vi "snapdragon_elka_quad.vi"() -> ()   [LabVIEW 2017]
uses:
  <vilib>/Instr/_visa.llb/VISA Flush IO Buffer Mask.ctl
  <vilib>/Instr/_visa.llb/VISA Configure Serial Port (Instr).vi
  <vilib>/Utility/file.llb/Write Delimited Spreadsheet (I64).vi
panel:
  in  "vio_yawki":i16=192
  in  "ixy_sens":i16=41
  in  "vio_yawkp":i16=2322
  in  "z_ki":i16=188
  out "base_thrust":i16(graph)
  in  "file path (dialog if empty) 2":path=path "C:/Users/Eric Solomon/Documents/elka/tests/sample_test.txt"
  in  "writte to file? 2":bool
  out "roll":i32(graph)
  out "thrust":i32(graph)
  out "z_error":i32(graph)
  out "y_error":i32(graph)
  in  "alt_kd":i16=-2
  in  "alt_kp":i16=-4
  in  "z_kp":i16=2330
  in  "z_kd":i16=70
  in  "vxy_sens":i16=26
  in  "xy_sens":i16=122
  in  "yawkd":i16=80
  in  "rollki":i16
  in  "rollkp":i16=2
  in  "Thrust Trim":i16(slide)=900 scale=-200.0..1500.0
  in  "Roll Trim":i16(slide) scale=-1000.0..1000.0
  in  "Pitch Trim":i16(slide) scale=-1000.0..1000.0
  in  "Yaw Trim":i16(slide) scale=-2000.0..2000.0
  out "appended array 2":u32[](array[numeric])=[11, 3, 255, 255, 3, 132, 0, 0, 0, 0, 0, 0]
  out "read buffer 2":string
  in  "STOP TRIM":bool
  out "read buffer 4":string
  out "appended array 4":u32[](array[numeric])=[15, 2, 255, 255, 0, 10, 0, 2, 0, 2, 255, 246, 255, 252, 255, 254]
  in  "Yaw_sens":i16=-10
  in  "Pitch_sens":i16=2
  in  "Roll_sens":i16=2
  in  "Thrust_sens":i16=10
  out "read buffer 3":string
  out "appended array 3":u32[](array[numeric])=[25, 1, 255, 255, 0, 2, 0, 0, 0, 40, 0, 2, 0, 0, 0, 40, 255, 176, 0, 15, 255, 248, 0, 7, 0, 5]
  in  "rollkd":i16=40
  in  "pitchki":i16
  in  "pitchkd":i16=40
  in  "pitchkp":i16=-2
  out "appended array":u32[](array[numeric])
  in  "channel4":i16
  in  "channel3":i16
  in  "channel2":i16
  in  "channel1":i16(slide) scale=0.0..2000.0
  out "read buffer":string
  out "pilot array":u8[](array[numeric])=[255, 247, 5, 220, 0, 15, 0, 115, 254, 40, 0, 0, 0, 0, 0, 0, 0, 0, 0, 0, 0, 0, 0, 0, 0, 0, 3, 132, 0, 2]
  out "GYRO X (deg/s)":i16(graph)=-9
  out "GYRO Y":i16(graph)=1500
  out "GYRO Z":i16(graph)=15
  out "Roll":i16(graph)=115
  out "Pitch":i16(graph)=-472
  out "x_error":i32(graph)
  out "Serial Settings:Number of Bytes at Serial Port":u32=32
  in  "XBEE STOP":bool
  in  "flow control 3":u16(ring) items=["None"=0, "XON/XOFF"=1, "RTS/CTS"=2, "DTR/DSR"=4]
  in  "stop bits 3":u16(ring)=10 items=["1.0"=10, "1.5"=15, "2.0"=20]
  in  "parity 3":u16(ring) items=["None", "Odd", "Even", "Mark", "Space"]
  in  "data bits 3":u16=8 min=5 max=8 step=1
  in  "VISA resource name 3":refnum<visa-resource-name>="COM7"
  in  "baud rate 3":u32=38400
  # "RECEIVE"
  # "GAINS"
  # "SENSITIVITY"
  # "Attitude Gains"
  # "Position Gains"
  # "-8"
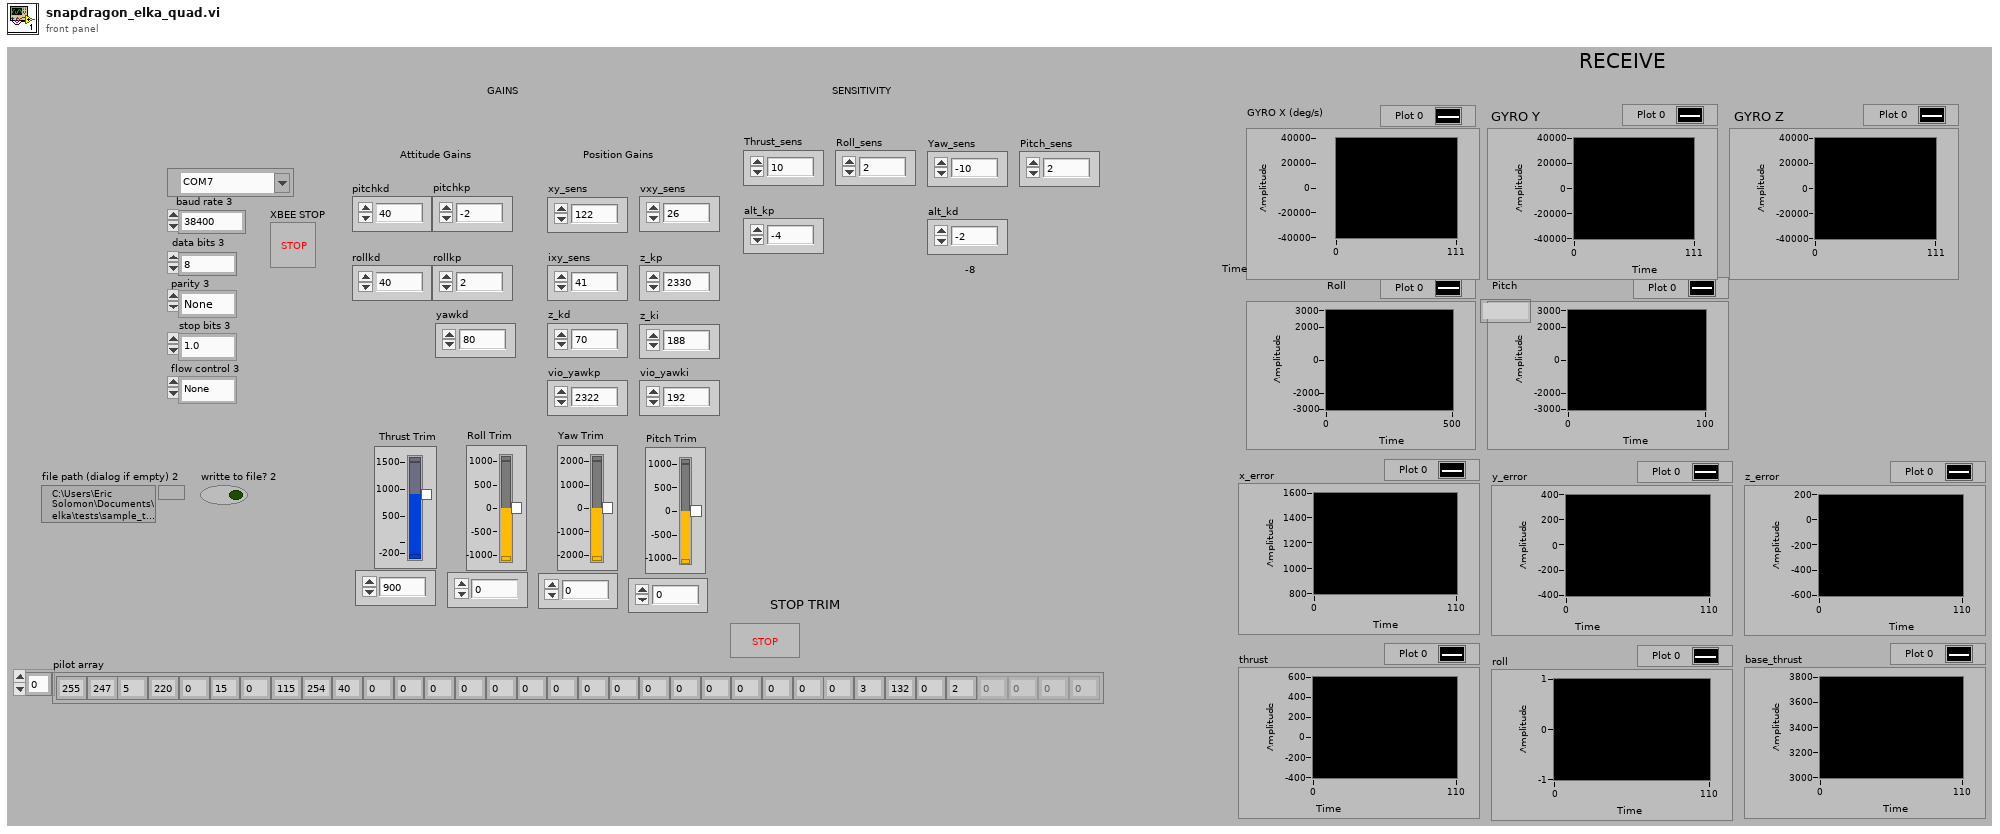
[diagram p1: front panel]
types:
  T1 = cluster{i32, i32, i32, i32, i32, i32, i32, i32, i32, i32, i32, i32, i32, i32, i32, i32}
  T2 = typedef "VISA Flush IO Buffer Mask.ctl" = u16
  T3 = cluster{i16, i16, i16, i16, i16, i32, i32, i32, i32, i32, i16, i32, i32, i32, i32, "millisecond timer value":u32}
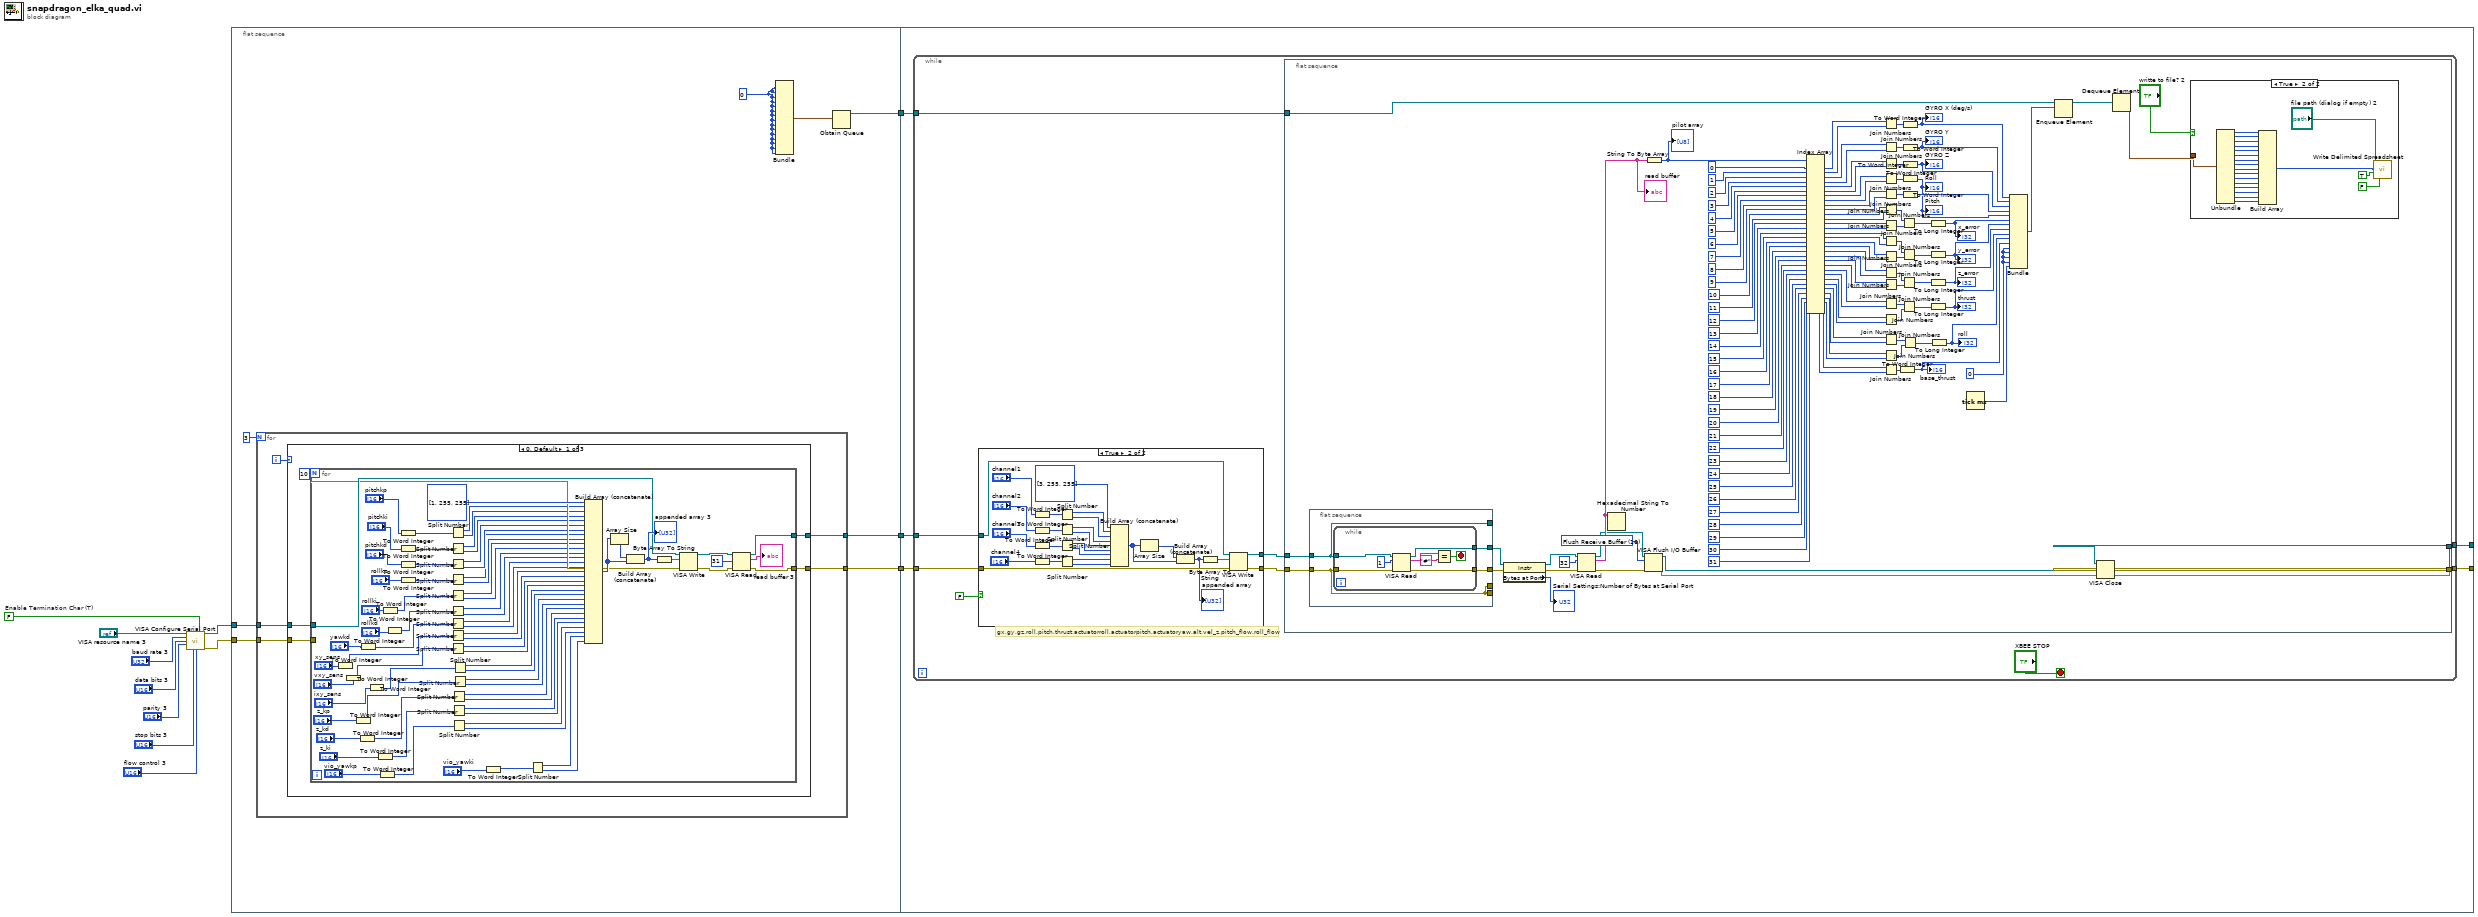
[diagram p0: block diagram]
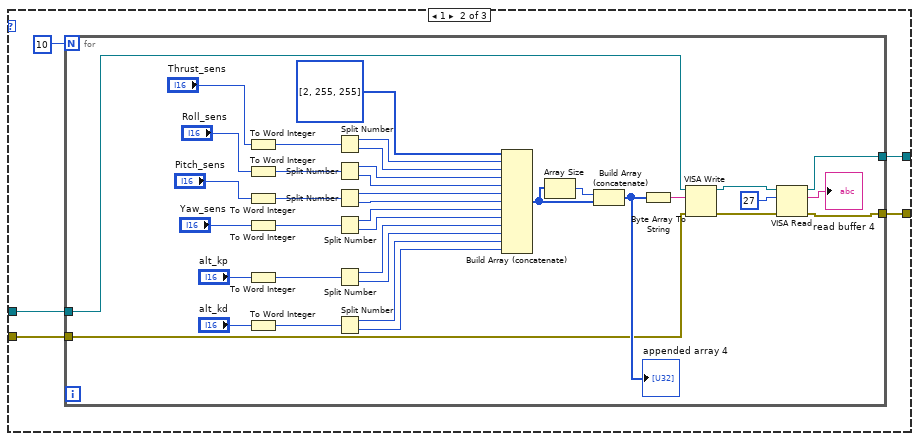
[diagram p2: hidden frame]
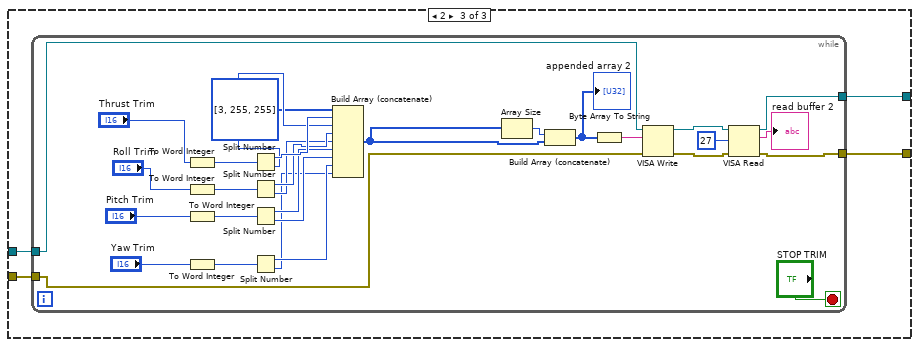
[diagram p3: hidden frame]
diagram:
  w11 = FALSE  # Enable Termination Char (T)
  n1 = call-poly "VISA Configure Serial Port"("VISA resource name"="VISA resource name 3", "Enable Termination\nChar (T)"=w11, "baud rate (9600)"="baud rate 3", "data bits (8)"="data bits 3", "parity (0:none)"="parity 3", "stop bits (10: 1 bit)"="stop bits 3", "flow control (0:none)"="flow control 3") -> ("VISA resource name out"=w6:refnum<visa-resource-name>, "error out"=w5:errorcluster)  [unwired: 1 in, 6 out]
  n2 = flat-sequence {
    tunnel: w5 -> [w21]
    tunnel: w6 -> [w22]
    tunnel: [w20] -> w4
    tunnel: [w19] -> w3
    tunnel: [w15] -> w1
    tunnel: [w186] -> w7
    tunnel: w4 -> [w185]
    tunnel: w3 -> [w184]
    tunnel: [w183] -> w2
    tunnel: w1 -> [w182]
    frame #0 {
      w16 = 0
      n3 = for {
        N: 3 -> [_]
        tunnel: w22 -> [w27]
        tunnel: [w25] -> w20
        tunnel: w21 -> [w26]
        tunnel: [w24] -> w19
        i -> [w23]
        n4 = case shown="0, Default" w23 {
          tunnel: w27 -> [w32 w110 w151]
          tunnel: w26 -> [w31 w107 w150]
          tunnel: [w30 w109 w149] -> w25
          tunnel: [w29 w108 w148] -> w24
          frame 0, Default {
            n5 = for {
              N: 10 -> [_]
              tunnel: w32 -> [w91]
              tunnel: [w89] -> w30
              tunnel: w31 -> [w90]
              tunnel: [w88] -> w29
              n6 = To Word Integer(number="xy_sens") -> (16bit integer=w72:i16)
              n7 = To Word Integer(number="vxy_sens") -> (16bit integer=w71:i16)
              n8 = To Word Integer(number="z_kp") -> (16bit integer=w70:i16)
              n9 = To Word Integer(number="z_kd") -> (16bit integer=w69:i16)
              n10 = To Word Integer(number="yawkd") -> (16bit integer=w84:i16)
              n11 = To Word Integer(number="ixy_sens") -> (16bit integer=w37:i16)
              n12 = To Word Integer(number="z_ki") -> (16bit integer=w58:i16)
              n13 = To Word Integer(number="vio_yawkp") -> (16bit integer=w57:i16)
              n14 = To Word Integer(number="rollki") -> (16bit integer=w86:i16)
              n15 = To Word Integer(number="rollkd") -> (16bit integer=w85:i16)
              n16 = To Word Integer(number="pitchkp") -> (16bit integer=w104:i16)
              n17 = To Word Integer(number="pitchki") -> (16bit integer=w103:i16)
              n18 = To Word Integer(number="pitchkd") -> (16bit integer=w102:i16)
              n19 = To Word Integer(number="rollkp") -> (16bit integer=w101:i16)
              n20 = Split Number(x=w104) -> (hi(x)=w52:u8, lo(x)=w51:u8)
              n21 = Split Number(x=w103) -> (hi(x)=w50:u8, lo(x)=w49:u8)
              n22 = Split Number(x=w102) -> (hi(x)=w48:u8, lo(x)=w47:u8)
              n23 = Split Number(x=w101) -> (hi(x)=w46:u8, lo(x)=w45:u8)
              n24 = Split Number(x=w86) -> (hi(x)=w44:u8, lo(x)=w43:u8)
              n25 = Split Number(x=w85) -> (hi(x)=w42:u8, lo(x)=w41:u8)
              n26 = Split Number(x=w84) -> (hi(x)=w83:u8, lo(x)=w82:u8)
              n27 = Split Number(x=w72) -> (hi(x)=w61:u8, lo(x)=w62:u8)
              n28 = Split Number(x=w71) -> (hi(x)=w63:u8, lo(x)=w64:u8)
              n29 = Split Number(x=w69) -> (hi(x)=w67:u8, lo(x)=w68:u8)
              n30 = Split Number(x=w57) -> (hi(x)=w54:u8, lo(x)=w53:u8)
              n31 = Split Number(x=w58) -> (hi(x)=w56:u8, lo(x)=w55:u8)
              n32 = Split Number(x=w37) -> (hi(x)=w39:u8, lo(x)=w38:u8)
              n33 = Split Number(x=w70) -> (hi(x)=w65:u8, lo(x)=w66:u8)
              n34 = To Word Integer(number="vio_yawki") -> (16bit integer=w34:i16)
              n35 = Split Number(x=w34) -> (hi(x)=w36:u8, lo(x)=w35:u8)
              n36 = Build Array (concatenate)(i32[] [1, 255, 255], w52, w51, w50, w49, w48, w47, w46, w45, w44, w43, w42, w41, w83, w82, w61, w62, w63, w64, w39, w38, w65, w66, w67, w68, w56, w55, w54, w53, w36, w35) -> (w98:i32[])
              n37 = Array Size(array=w98) -> (size(s)=w99:i32)
              n38 = Build Array (concatenate)(w99, w98) -> (w97:i32[])
              "appended array 3" <- w97
              n39 = Byte Array To String(unsigned byte array=w97) -> (string=w100:string)
              n40 = VISA Write(VISA resource name=w91, write buffer=w100, error in (no error)=w90) -> (VISA resource name out=w95:refnum<visa-resource-name>, error out=w94:errorcluster)  [unwired: 1 out]
              n41 = VISA Read(VISA resource name=w95, byte count=u32 31, error in (no error)=w94) -> (VISA resource name out=w89:refnum<visa-resource-name>, read buffer=→"read buffer 3":string, error out=w88:errorcluster)  [unwired: 1 out]
            }
          }
          frame 1 {
            n42 = for {
              N: 10 -> [_]
              tunnel: w110 -> [w122]
              tunnel: [w121] -> w109
              tunnel: w107 -> [w119]
              tunnel: [w120] -> w108
              n43 = To Word Integer(number="Thrust_sens") -> (16bit integer=w146:i16)
              n44 = To Word Integer(number="Roll_sens") -> (16bit integer=w144:i16)
              n45 = To Word Integer(number="Pitch_sens") -> (16bit integer=w142:i16)
              n46 = To Word Integer(number="Yaw_sens") -> (16bit integer=w140:i16)
              n47 = To Word Integer(number="alt_kp") -> (16bit integer=w116:i16)
              n48 = To Word Integer(number="alt_kd") -> (16bit integer=w115:i16)
              n49 = Split Number(x=w146) -> (hi(x)=w139:u8, lo(x)=w138:u8)
              n50 = Split Number(x=w144) -> (hi(x)=w137:u8, lo(x)=w136:u8)
              n51 = Split Number(x=w142) -> (hi(x)=w135:u8, lo(x)=w134:u8)
              n52 = Split Number(x=w140) -> (hi(x)=w133:u8, lo(x)=w132:u8)
              n53 = Split Number(x=w116) -> (hi(x)=w114:u8, lo(x)=w113:u8)
              n54 = Split Number(x=w115) -> (hi(x)=w112:u8, lo(x)=w111:u8)
              n55 = Build Array (concatenate)(i32[] [2, 255, 255], w139, w138, w137, w136, w135, w134, w133, w132, w114, w113, w112, w111) -> (w129:i32[])
              n56 = Array Size(array=w129) -> (size(s)=w130:i32)
              n57 = Build Array (concatenate)(w130, w129) -> (w128:i32[])
              "appended array 4" <- w128
              n58 = Byte Array To String(unsigned byte array=w128) -> (string=w131:string)
              n59 = VISA Write(VISA resource name=w122, write buffer=w131, error in (no error)=w119) -> (VISA resource name out=w126:refnum<visa-resource-name>, error out=w125:errorcluster)  [unwired: 1 out]
              n60 = VISA Read(VISA resource name=w126, byte count=u32 27, error in (no error)=w125) -> (VISA resource name out=w121:refnum<visa-resource-name>, read buffer=→"read buffer 4":string, error out=w120:errorcluster)  [unwired: 1 out]
            }
          }
          frame 2 {
            n61 = while {
              tunnel: w151 -> [w181]
              tunnel: [w179] -> w149
              tunnel: w150 -> [w180]
              tunnel: [w178] -> w148
              stop <- "STOP TRIM" stop-if-true
              n62 = To Word Integer(number="Thrust Trim") -> (16bit integer=w176:i16)
              n63 = To Word Integer(number="Roll Trim") -> (16bit integer=w174:i16)
              n64 = To Word Integer(number="Pitch Trim") -> (16bit integer=w172:i16)
              n65 = To Word Integer(number="Yaw Trim") -> (16bit integer=w170:i16)
              n66 = Split Number(x=w176) -> (hi(x)=w169:u8, lo(x)=w168:u8)
              n67 = Split Number(x=w174) -> (hi(x)=w167:u8, lo(x)=w166:u8)
              n68 = Split Number(x=w172) -> (hi(x)=w165:u8, lo(x)=w164:u8)
              n69 = Split Number(x=w170) -> (hi(x)=w163:u8, lo(x)=w162:u8)
              n70 = Build Array (concatenate)(i32[] [3, 255, 255], w169, w168, w167, w166, w165, w164, w163, w162) -> (w159:i32[])
              n71 = Array Size(array=w159) -> (size(s)=w160:i32)
              n72 = Build Array (concatenate)(w160, w159) -> (w158:i32[])
              "appended array 2" <- w158
              n73 = Byte Array To String(unsigned byte array=w158) -> (string=w161:string)
              n74 = VISA Write(VISA resource name=w181, write buffer=w161, error in (no error)=w180) -> (VISA resource name out=w156:refnum<visa-resource-name>, error out=w155:errorcluster)  [unwired: 1 out]
              n75 = VISA Read(VISA resource name=w156, byte count=u32 27, error in (no error)=w155) -> (VISA resource name out=w179:refnum<visa-resource-name>, read buffer=→"read buffer 2":string, error out=w178:errorcluster)  [unwired: 1 out]
            }
          }
        }
      }
      n76 = Bundle(w16, w16, w16, w16, w16, w16, w16, w16, w16, w16, w16, w16, w16, w16, w16, w16) -> (w17:T1)  [unwired: 1 in]
      n77 = Obtain Queue(element data type=w17) -> (queue out=w15:refnum<queue>)  [unwired: 4 in, 2 out]
    }
    frame #1 {
      n78 = while {
        tunnel: w184 -> [w192]
        tunnel: w185 -> [w194]
        tunnel: [w195] -> w186
        tunnel: [w189] -> w183
        tunnel: w182 -> [w188]
        stop <- "XBEE STOP" stop-if-true
        # "gx,gy,gz,roll,pitch,thrust,actuatorroll,actuatorpitch,actuatoryaw,alt,vel_z,pitch_flow,roll_flow"
        n79 = case shown="True" FALSE {
          tunnel: w192 -> [w347 w372]
          tunnel: w194 -> [w348 w373]
          tunnel: [w348 w371] -> w193
          tunnel: [w347 w370] -> w191
          frame False {
          }
          frame True {
            n80 = To Word Integer(number="channel1") -> (16bit integer=w368:i16)
            n81 = To Word Integer(number="channel2") -> (16bit integer=w366:i16)
            n82 = To Word Integer(number="channel3") -> (16bit integer=w364:i16)
            n83 = To Word Integer(number="channel4") -> (16bit integer=w362:i16)
            n84 = Split Number(x=w368) -> (hi(x)=w361:u8, lo(x)=w360:u8)
            n85 = Split Number(x=w366) -> (hi(x)=w359:u8, lo(x)=w358:u8)
            n86 = Split Number(x=w364) -> (hi(x)=w357:u8, lo(x)=w356:u8)
            n87 = Split Number(x=w362) -> (hi(x)=w355:u8, lo(x)=w354:u8)
            n88 = Build Array (concatenate)(i32[] [3, 255, 255], w361, w360, w359, w358, w357, w356, w355, w354) -> (w351:i32[])
            n89 = Array Size(array=w351) -> (size(s)=w352:i32)
            n90 = Build Array (concatenate)(w352, w351) -> (w350:i32[])
            "appended array" <- w350
            n91 = Byte Array To String(unsigned byte array=w350) -> (string=w353:string)
            n92 = VISA Write(VISA resource name=w373, write buffer=w353, error in (no error)=w372) -> (VISA resource name out=w371:refnum<visa-resource-name>, error out=w370:errorcluster)  [unwired: 1 out]
          }
        }
        n93 = flat-sequence {
          tunnel: [w266] -> w189
          tunnel: [w265] -> w195
          tunnel: w193 -> [w262]
          tunnel: w191 -> [w261]
          tunnel: w188 -> [w205]
          frame #0 {
            w207 = 0
            w310 = T2 16 items=["Flush Receive Buffer"=16, "Write Transmit Buffer to Device"=32, "Flush Receive Buffer (No I/O)"=64, "Flush Transmit Buffer"=128] ("Mask")
            n94 = flat-sequence {
              tunnel: [w338] -> w313
              tunnel: [w337] -> w312
              tunnel: [w335] -> _
              tunnel: [w336] -> _
              tunnel: [w336] -> _
              tunnel: w261 -> [w336]
              tunnel: w262 -> [w335]
              frame #0 {
                n95 = while {
                  tunnel: [w344] -> w338
                  tunnel: [w343] -> w337
                  tunnel: w335 -> [w342]
                  tunnel: w336 -> [w341]
                  stop <- w345 stop-if-true
                  n96 = VISA Read(VISA resource name=w342, byte count=u32 1, error in (no error)=w341) -> (VISA resource name out=w344:refnum<visa-resource-name>, read buffer=w340:string, error out=w343:errorcluster)  [unwired: 1 out]
                  n97 = Equal?(x=w340, y="#") -> (x = y?=w345:bool)
                }
              }
            }
            n98 = property class="Instr"(reference=w313, error in=w312) -> (reference out=w268:refnum<visa-resource-name>, error out=w267:errorcluster, "Bytes at Port"=→"Serial Settings:Number of Bytes at Serial Port":u32)
            n99 = VISA Read(VISA resource name=w268, byte count=u32 32, error in (no error)=w267) -> (VISA resource name out=w309:refnum<visa-resource-name>, read buffer=w311:string, error out=w308:errorcluster)  [unwired: 1 out]
            "read buffer" <- w311
            n100 = Hexadecimal String To Number(string=w311) -> ()  [unwired: 2 in, 2 out]
            n101 = VISA Flush I/O Buffer(VISA resource name=w309, mask (16)=w310, error in (no error)=w308) -> (VISA resource name out=w266:refnum<visa-resource-name>, error out=w265:errorcluster)
            n102 = String To Byte Array(string=w311) -> (unsigned byte array=w260:u8[])
            "pilot array" <- w260
            n103 = Index Array(array=w260, index #1=0 ("index"), index #2=1 ("index"), index #3=2 ("index"), index #4=3 ("index"), index #5=4 ("index"), index #6=5 ("index"), index #7=6 ("index"), index #8=7 ("index"), index #9=8 ("index"), index #10=9 ("index"), index #11=10 ("index"), index #12=11 ("index"), index #13=12 ("index"), index #14=13 ("index"), index #15=14 ("index"), index #16=15 ("index"), index #17=16 ("index"), index #18=17 ("index"), index #19=18 ("index"), index #20=19 ("index"), index #21=20 ("index"), index #22=21 ("index"), index #23=22 ("index"), index #24=23 ("index"), index #25=24 ("index"), index #26=25 ("index"), index #27=26 ("index"), index #28=27 ("index"), index #29=28 ("index"), index #30=29 ("index"), index #31=30 ("index"), index #32=31 ("index")) -> (element #1=w307:u8, element #2=w306:u8, element #3=w293:u8, element #4=w292:u8, element #5=w291:u8, element #6=w290:u8, element #7=w289:u8, element #8=w288:u8, element #9=w287:u8, element #10=w286:u8, element #11=w235:u8, element #12=w234:u8, element #13=w233:u8, element #14=w232:u8, element #15=w231:u8, element #16=w230:u8, element #17=w229:u8, element #18=w228:u8, element #19=w227:u8, element #20=w226:u8, element #21=w225:u8, element #22=w224:u8, element #23=w223:u8, element #24=w222:u8, element #25=w221:u8, element #26=w220:u8, element #27=w212:u8, element #28=w211:u8, element #29=w210:u8, element #30=w209:u8, element #31=w199:u8, element #32=w198:u8)
            n104 = Join Numbers(hi=w307, lo=w306) -> ((hi.lo)=w255:u16)
            n105 = Join Numbers(hi=w293, lo=w292) -> ((hi.lo)=w254:u16)
            n106 = Join Numbers(hi=w291, lo=w290) -> ((hi.lo)=w285:u16)
            n107 = Join Numbers(hi=w289, lo=w288) -> ((hi.lo)=w284:u16)
            n108 = Join Numbers(hi=w287, lo=w286) -> ((hi.lo)=w283:u16)
            n109 = Join Numbers(hi=w235, lo=w234) -> ((hi.lo)=w248:u16)
            n110 = Join Numbers(hi=w233, lo=w232) -> ((hi.lo)=w247:u16)
            n111 = Join Numbers(hi=w231, lo=w230) -> ((hi.lo)=w245:u16)
            n112 = Join Numbers(hi=w229, lo=w228) -> ((hi.lo)=w244:u16)
            n113 = Join Numbers(hi=w227, lo=w226) -> ((hi.lo)=w242:u16)
            n114 = Join Numbers(hi=w225, lo=w224) -> ((hi.lo)=w241:u16)
            n115 = Join Numbers(hi=w223, lo=w222) -> ((hi.lo)=w239:u16)
            n116 = Join Numbers(hi=w221, lo=w220) -> ((hi.lo)=w238:u16)
            n117 = Join Numbers(hi=w199, lo=w198) -> ((hi.lo)=w197:u16)
            n118 = Join Numbers(hi=w212, lo=w211) -> ((hi.lo)=w215:u16)
            n119 = Join Numbers(hi=w210, lo=w209) -> ((hi.lo)=w214:u16)
            n120 = To Word Integer(number=w197) -> (16bit integer=w196:i16)
            "base_thrust" <- w196
            n121 = Join Numbers(hi=w248, lo=w247) -> ((hi.lo)=w246:u32)
            n122 = Join Numbers(hi=w245, lo=w244) -> ((hi.lo)=w243:u32)
            n123 = Join Numbers(hi=w242, lo=w241) -> ((hi.lo)=w240:u32)
            n124 = Join Numbers(hi=w239, lo=w238) -> ((hi.lo)=w237:u32)
            n125 = To Word Integer(number=w255) -> (16bit integer=w253:i16)
            "GYRO X (deg/s)" <- w253
            n126 = To Word Integer(number=w254) -> (16bit integer=w252:i16)
            "GYRO Y" <- w252
            n127 = To Word Integer(number=w285) -> (16bit integer=w251:i16)
            "GYRO Z" <- w251
            n128 = To Word Integer(number=w284) -> (16bit integer=w250:i16)
            "Roll" <- w250
            n129 = To Word Integer(number=w283) -> (16bit integer=w249:i16)
            "Pitch" <- w249
            n130 = Join Numbers(hi=w215, lo=w214) -> ((hi.lo)=w213:u32)
            n131 = To Long Integer(number=w246) -> (32bit integer=w219:i32)
            "x_error" <- w219
            n132 = To Long Integer(number=w243) -> (32bit integer=w218:i32)
            "y_error" <- w218
            n133 = To Long Integer(number=w240) -> (32bit integer=w217:i32)
            "z_error" <- w217
            n134 = To Long Integer(number=w237) -> (32bit integer=w216:i32)
            "thrust" <- w216
            n135 = To Long Integer(number=w213) -> (32bit integer=w208:i32)
            "roll" <- w208
            n136 = Tick Count (ms)() -> (millisecond timer value=w236:u32)
            n137 = Bundle(w253, w252, w251, w250, w249, w219, w218, w217, w216, w208, w196, w207, w207, w207, w207, "millisecond timer value"=w236) -> (w206:T3)  [unwired: 1 in]
            n138 = Enqueue Element(queue=w205, element=w206) -> (queue out=w202:refnum<queue>)  [unwired: 2 in, 2 out]
            n139 = Dequeue Element(queue=w202) -> (element=w204:T1)  [unwired: 2 in, 3 out]
            n140 = case shown="True" "writte to file? 2" {
              tunnel: w204 -> [_ w333]
              frame False {
              }
              frame True {
                n141 = Unbundle(w333) -> (w332:i32, w331:i32, w330:i32, w329:i32, w328:i32, w327:i32, w326:i32, w325:i32, w324:i32, w323:i32, w321:i32, w320:i32, w319:i32, w318:i32, w317:i32, w322:i32)
                n142 = Build Array(w332, w331, w330, w329, w328, w327, w326, w325, w324, w323, w321, w320, w319, w318, w317, w322) -> (w316:i32[])
                n143 = call-poly <vilib>:"Write Delimited Spreadsheet.vi"("file path (dialog if empty)"="file path (dialog if empty) 2", "1D data"=w316, "append to file? (new file:F)"=TRUE, "transpose? (no:F)"=FALSE) -> ()  [unwired: 10 in, 2 out]
              }
            }
          }
        }
      }
    }
  }
  n144 = VISA Close(VISA resource name=w2, error in (no error)=w7) -> ()  [unwired: 1 out]
